vi "PIM Convert 1.2-3 to 2.0.vi"(0 "PIM 1.2/3 Test Parameters":T2={"Stimulus"={"C1 Pwr dBm"=0.0, "C2 Pwr dBm"=0.0, "Power Units"=enum."dBm", "Meas Type"=enum."Fixed Pair", "C1 Fixed MHz"=0.0, "C2 Fixed MHz"=0.0, "Swept Freq Step"=0}, "Measure"={"IM Order"=0, "Direction"=0, "Averaging"=0, "ALC ON?"=FALSE, "Peak Hold?"=FALSE, "Peak last N"=0, "Ref Level dBm"=0.0, "Ref Units"=enum."dBm", "Num Samples"=0, "Sample units"=enum."Sample(s)", "Update Rate (s)"=0.0}, "Display"={"Power Scale"={"yRange_min"=0, "yRange_max"=0}, "xRange_span"=0}} {"Stimulus"."C2 Fixed MHz" min=-200.0 max=0.0 step=0.2 format="%.1f"; "Stimulus"."C1 Fixed MHz" min=-200.0 max=0.0 step=0.2 format="%.1f"; "Stimulus"."Swept Freq Step" items=[".2", ".4", "1.0", "2.0"]; "Measure"."IM Order" items=["3rd", "5th", "7th", "9th", "11th", "13th", "15th", "17th", "19th", "21st", "23rd", "25th", "27th", "29th", "31st", "33rd"]; "Measure"."Direction" items=["Reverse", "Forward", "Auxiliary"]; "Measure"."Averaging" items=["None", "Minimum", "Normal", "High", "Maximum"]}) -> (2 "PIM 2.0 Test Parameters":T1={"Stimulus"={"C1 Pwr dBm"=0.0, "C2 Pwr dBm"=0.0, "Power Units"=enum."dBm", "Meas Type"=enum."Time", "C1 Freq MHz"=0.0, "C2 Freq MHz"=0.0, "Swept Freq Step"=0}, "Measure"={"IM Order"=0, "Direction"=0, "Averaging"=1, "ALC ON?"=TRUE, "Peak Hold?"=TRUE, "Peak last N"=1, "Ref Level dBm"=-100.0, "Ref Units"=enum."dBm", "Num Samples"=1, "Sample units"=enum."Sample(s)", "Update Rate (s)"=0.0, "DUT PORT"=enum."Port 1"}, "Display"={"Power Scale"={"yRange_min"=-160, "yRange_max"=-60}, "xRange_span"=5}} {"Stimulus"."Swept Freq Step" items=[".2", ".4", "1.0", "2.0"]; "Measure"."Averaging" items=["None", "Minimum", "Normal", "High", "Maximum"]; "Measure"."Direction" items=["Reverse", "Forward", "Auxiliary"]; "Measure"."IM Order" items=["3rd", "5th", "7th", "9th", "11th", "13th", "15th", "17th", "19th", "21st", "23rd", "25th", "27th", "29th", "31st", "33rd"]})   [LabVIEW 2011]
uses:
  TypeDefs/PIM Test Parameters v1.2-1.3.ctl
  SI.LIB/PIM.LIB/HW IO/IMOrder.ctl
  SI.LIB/PIM.LIB/HW IO/MeasMode.ctl
  SI.LIB/PIM.LIB/HW IO/HW Averaging.ctl
  TypeDefs/PIM Meas Units.ctl
  TypeDefs/PIM Display Parameters.ctl
  TypeDefs/PIM Test Parameters v2.0-6.1.ctl
  SI.LIB/PIM.LIB/HW IO/DUTport.ctl
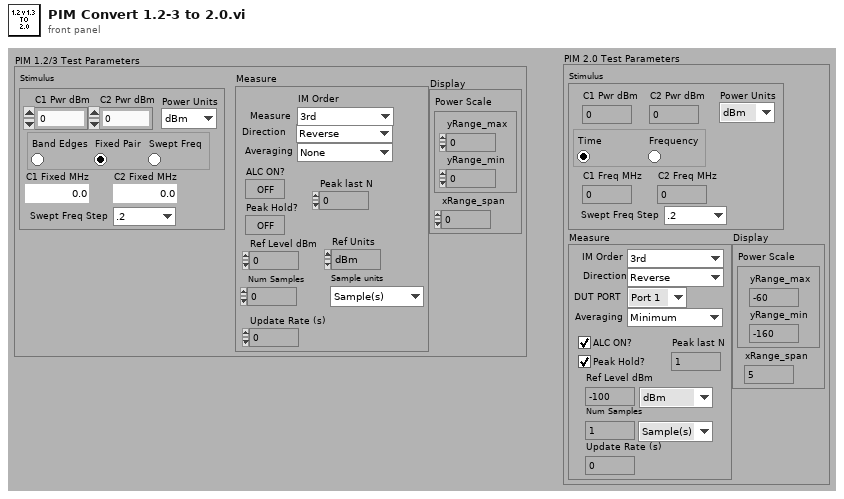
[diagram p1: front panel]
types:
  T1 = typedef "PIM Test Parameters v2.0-6.1.ctl" = cluster{"Stimulus":cluster{"C1 Pwr dBm":dbl, "C2 Pwr dBm":dbl, "Power Units":enum16{"dBm", "Watts"}, "Meas Type":enum32{"Time", "Frequency"}, "C1 Freq MHz":dbl, "C2 Freq MHz":dbl, "Swept Freq Step":u16}, "Measure":cluster{"IM Order":u8, "Direction":u16, "Averaging":u16, "ALC ON?":bool, "Peak Hold?":bool, "Peak last N":u32, "Ref Level dBm":dbl, "Ref Units":enum16{"dBm", "dBc"}, "Num Samples":u32, "Sample units":enum16{"Sample(s)", "Second(s)", "Sweep(s)"}, "Update Rate (s)":dbl, "DUT PORT":enum16{"Port 1", "Port 2"}}, "Display":cluster{"Power Scale":cluster{"yRange_min":i32, "yRange_max":i32}, "xRange_span":u32}}
  T2 = typedef "PIM Test Parameters v1.2-1.3.ctl" = cluster{"Stimulus":cluster{"C1 Pwr dBm":dbl, "C2 Pwr dBm":dbl, "Power Units":enum16{"dBm", "Watts"}, "Meas Type":enum32{"Band Edges", "Fixed Pair", "Swept Freq"}, "C1 Fixed MHz":dbl, "C2 Fixed MHz":dbl, "Swept Freq Step":u16}, "Measure":cluster{"IM Order":T3, "Direction":T4, "Averaging":T5, "ALC ON?":bool, "Peak Hold?":bool, "Peak last N":u32, "Ref Level dBm":dbl, "Ref Units":enum16{"dBm", "dBc"}, "Num Samples":u32, "Sample units":T6, "Update Rate (s)":dbl}, "Display":T7}
  T3 = typedef "IMOrder.ctl" = u8
  T4 = typedef "MeasMode.ctl" = u16
  T5 = typedef "HW Averaging.ctl" = u16
  T6 = typedef "PIM Meas Units.ctl" = enum16{"Sample(s)", "Second(s)", "Sweep(s)"}
  T7 = typedef "PIM Display Parameters.ctl" = cluster{"Power Scale":cluster{"yRange_min":i32, "yRange_max":i32}, "xRange_span":u32}
  T8 = typedef "DUTport.ctl" = enum16{"Port 1", "Port 2"}
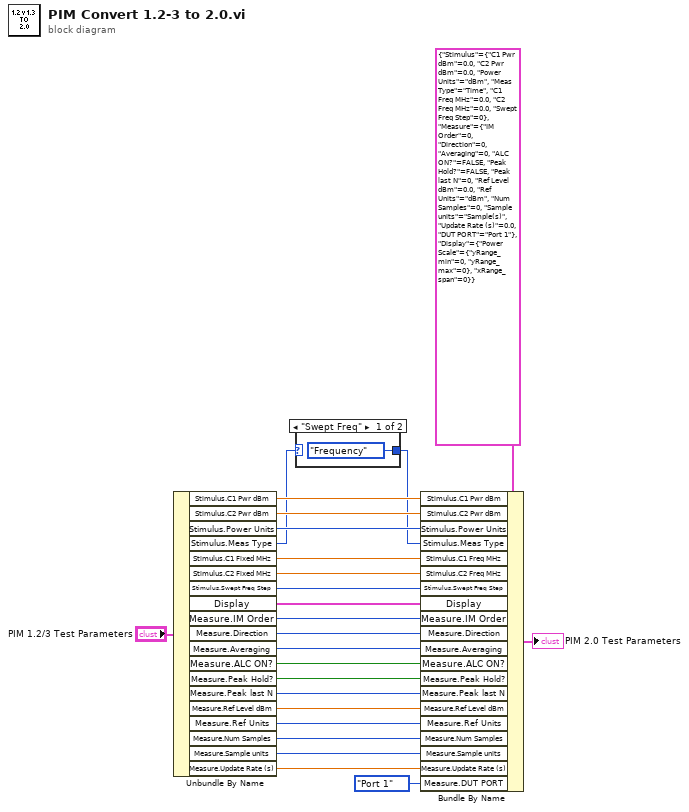
[diagram p0: block diagram]
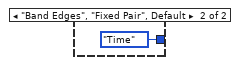
[diagram p2: hidden frame]
diagram:
  n1 = Unbundle By Name("PIM 1.2/3 Test Parameters") -> ("Stimulus.C1 Pwr dBm"=w3:dbl, "Stimulus.C2 Pwr dBm"=w4:dbl, "Stimulus.Power Units"=w5:enum16{"dBm", "Watts"}, "Stimulus.Meas Type"=w2:enum32{"Band Edges", "Fixed Pair", "Swept Freq"}, "Stimulus.C1 Fixed MHz"=w6:dbl, "Stimulus.C2 Fixed MHz"=w7:dbl, "Stimulus.Swept Freq Step"=w8:u16, "Display"=w24:T7, "Measure.IM Order"=w21:T3, "Measure.Direction"=w20:T4, "Measure.Averaging"=w19:T5, "Measure.ALC ON?"=w18:bool, "Measure.Peak Hold?"=w17:bool, "Measure.Peak last N"=w16:u32, "Measure.Ref Level dBm"=w15:dbl, "Measure.Ref Units"=w14:enum16{"dBm", "dBc"}, "Measure.Num Samples"=w13:u32, "Measure.Sample units"=w12:T6, "Measure.Update Rate (s)"=w11:dbl)
  n2 = case shown="\"Swept Freq\"" w2 {
    tunnel: [enum32{"Time", "Frequency"}."Frequency" ("Stimulus.Meas Type") enum32{"Time", "Frequency"}."Time" ("Stimulus.Meas Type")] -> w1
    frame "Swept Freq" {
    }
    frame "Band Edges", "Fixed Pair", Default {
    }
  }
  n3 = Bundle By Name(cluster=T1 {"Stimulus"={"C1 Pwr dBm"=0.0, "C2 Pwr dBm"=0.0, "Power Units"=enum."dBm", "Meas Type"=enum."Time", "C1 Freq MHz"=0.0, "C2 Freq MHz"=0.0, "Swept Freq Step"=0}, "Measure"={"IM Order"=0, "Direction"=0, "Averaging"=0, "ALC ON?"=FALSE, "Peak Hold?"=FALSE, "Peak last N"=0, "Ref Level dBm"=0.0, "Ref Units"=enum."dBm", "Num Samples"=0, "Sample units"=enum."Sample(s)", "Update Rate (s)"=0.0, "DUT PORT"=enum."Port 1"}, "Display"={"Power Scale"={"yRange_min"=0, "yRange_max"=0}, "xRange_span"=0}} ("PIM 1.1 Test Parameters"), "Stimulus.C1 Pwr dBm"=w3, "Stimulus.C2 Pwr dBm"=w4, "Stimulus.Power Units"=w5, "Stimulus.Meas Type"=w1, "Stimulus.C1 Freq MHz"=w6, "Stimulus.C2 Freq MHz"=w7, "Stimulus.Swept Freq Step"=w8, "Display"=w24, "Measure.IM Order"=w21, "Measure.Direction"=w20, "Measure.Averaging"=w19, "Measure.ALC ON?"=w18, "Measure.Peak Hold?"=w17, "Measure.Peak last N"=w16, "Measure.Ref Level dBm"=w15, "Measure.Ref Units"=w14, "Measure.Num Samples"=w13, "Measure.Sample units"=w12, "Measure.Update Rate (s)"=w11, "Measure.DUT PORT"=DUTport."Port 1") -> (→"PIM 2.0 Test Parameters":T1)
